vi "Display.vi"(0 "Pressure":dbl=666.0, 1 "InsightMode":T3, 2 "LineOneInfo":T2, 3 "LineTwoInfo":T1, 5 "Temp":string="666", 7 "Angle":dbl=666.0, 9 "Distance":dbl=666.0) -> ()   [LabVIEW 2013]
uses:
  InsightMode.ctl
  LineOneInfo.ctl
  LineTwoInfo.ctl
  <vilib>/Rock Robotics/SystemInterfaces/Typedef/FPGA_TypedefDigitalModule.ctl
  Insight Float Package.vi
  Insight String Package.vi
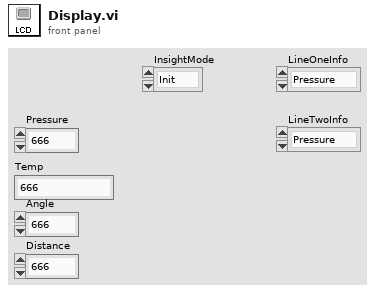
[diagram p1: front panel]
types:
  T1 = typedef "LineTwoInfo.ctl" = enum16{"Pressure", "Temperatue", "Angle", "Distance"}
  T2 = typedef "LineOneInfo.ctl" = enum16{"Pressure", "Temperature", "Angle", "Distance"}
  T3 = typedef "InsightMode.ctl" = enum16{"Init", "Write", "Display", "Disable"}
  T4 = typedef "FPGA_TypedefDigitalModule.ctl" = enum16{"Digital Module 1", "Digital Module 2"}
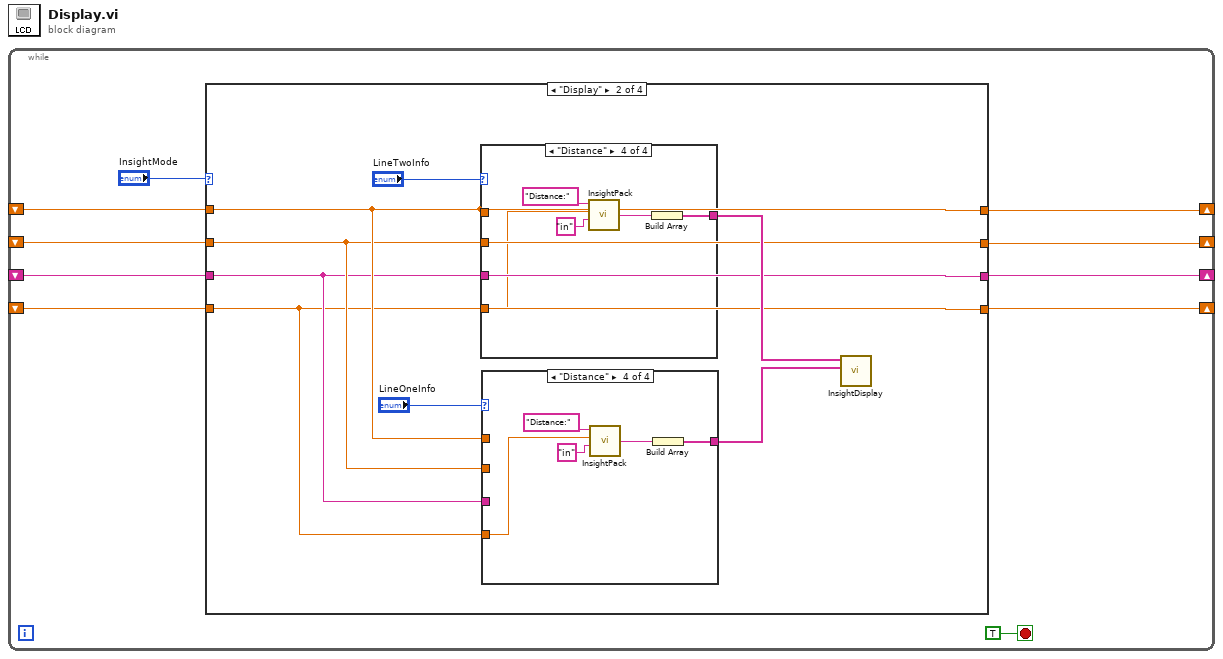
[diagram p0: block diagram]
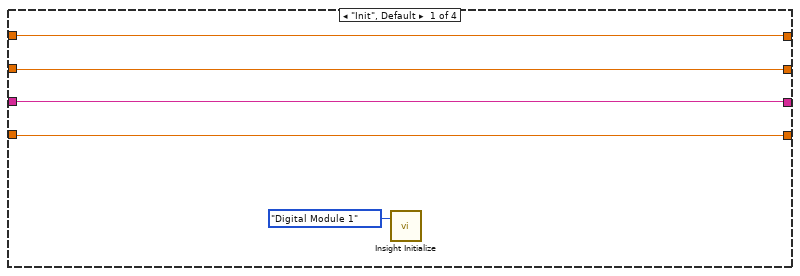
[diagram p2: hidden frame]
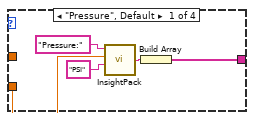
[diagram p3: hidden frame]
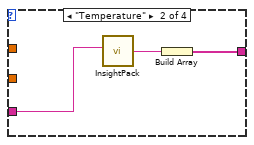
[diagram p4: hidden frame]
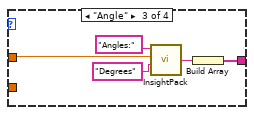
[diagram p5: hidden frame]
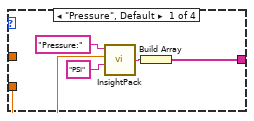
[diagram p6: hidden frame]
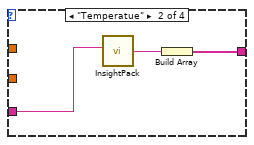
[diagram p7: hidden frame]
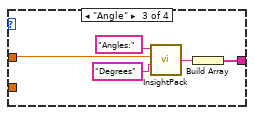
[diagram p8: hidden frame]
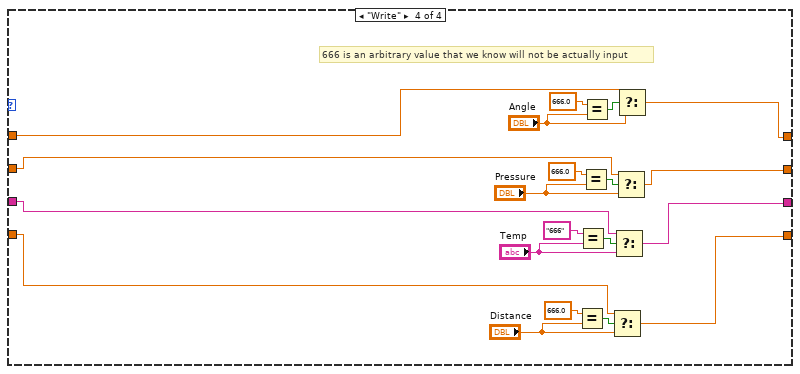
[diagram p10: hidden frame]
diagram:
  n1 = while {
    shift-right: [w6] -> _
    shift-left: _ -> [w5]
    shift-right: [w7] -> _
    shift-left: _ -> [w4]
    shift-right: [w8] -> _
    shift-left: _ -> [w2]
    shift-right: [w9] -> _
    shift-left: _ -> [w3]
    stop <- TRUE stop-if-true
    n2 = case shown="\"Display\"" "InsightMode" {
      tunnel: [w11 w19 w63 w83] -> w6
      tunnel: [w12 w18 w62 w79] -> w7
      tunnel: [w13 w17 w61 w69] -> w8
      tunnel: [w14 w16 w60 w74] -> w9
      tunnel: w5 -> [w11 w19 w63 w82]
      tunnel: w4 -> [w12 w18 w62 w78]
      tunnel: w2 -> [w13 w17 w61 w68]
      tunnel: w3 -> [w14 w16 w60 w73]
      frame "Init", Default {
        n3 = call "Insight Initialize.vi"("Digital Module"=FPGA_TypedefDigitalModule."Digital Module 1") -> ()  [unwired: 2 in]
      }
      frame "Display" {
        n4 = case shown="\"Distance\"" "LineTwoInfo" {
          tunnel: w19 -> [_ _ w52 _]
          tunnel: [w46 w49 w54 w56] -> w20
          tunnel: w18 -> [w44 _ _ _]
          tunnel: w17 -> [_ w48 _ _]
          tunnel: w16 -> [_ _ _ w59]
          frame "Pressure", Default {
            n5 = call-poly "InsightPack.vi"("Footer"="PSI", "Float"=w44, "Header"="Pressure:") -> ("resulting string"=w42:string)  [unwired: 1 in]
            n6 = Build Array(w42) -> (w46:string[])
          }
          frame "Temperatue" {
            n7 = call-poly "InsightPack.vi"("String"=w48) -> ("resulting string"=w47:string)  [unwired: 3 in]
            n8 = Build Array(w47) -> (w49:string[])
          }
          frame "Angle" {
            n9 = call-poly "InsightPack.vi"("Footer"="Degrees", "Float"=w52, "Header"="Angles:") -> ("resulting string"=w53:string)  [unwired: 1 in]
            n10 = Build Array(w53) -> (w54:string[])
          }
          frame "Distance" {
            n11 = call-poly "InsightPack.vi"("Footer"="in", "Float"=w59, "Header"="Distance:") -> ("resulting string"=w55:string)  [unwired: 1 in]
            n12 = Build Array(w55) -> (w56:string[])
          }
        }
        n13 = case shown="\"Distance\"" "LineOneInfo" {
          tunnel: w19 -> [_ _ w34 _]
          tunnel: [w28 w31 w36 w38] -> w21
          tunnel: w18 -> [w26 _ _ _]
          tunnel: w17 -> [_ w30 _ _]
          tunnel: w16 -> [_ _ _ w41]
          frame "Pressure", Default {
            n14 = call-poly "InsightPack.vi"("Footer"="PSI", "Float"=w26, "Header"="Pressure:") -> ("resulting string"=w24:string)  [unwired: 1 in]
            n15 = Build Array(w24) -> (w28:string[])
          }
          frame "Temperature" {
            n16 = call-poly "InsightPack.vi"("String"=w30) -> ("resulting string"=w29:string)  [unwired: 3 in]
            n17 = Build Array(w29) -> (w31:string[])
          }
          frame "Angle" {
            n18 = call-poly "InsightPack.vi"("Footer"="Degrees", "Float"=w34, "Header"="Angles:") -> ("resulting string"=w35:string)  [unwired: 1 in]
            n19 = Build Array(w35) -> (w36:string[])
          }
          frame "Distance" {
            n20 = call-poly "InsightPack.vi"("Footer"="in", "Float"=w41, "Header"="Distance:") -> ("resulting string"=w37:string)  [unwired: 1 in]
            n21 = Build Array(w37) -> (w38:string[])
          }
        }
        n22 = call "InsightDisplay.vi"("Zone 2 Data"=w21, "Zone 1 Data"=w20) -> ()  [unwired: 10 in]
      }
      frame "Disable" {
      }
      frame "Write" {
        # "666 is an arbitrary value that we know will not be actually input"
        n23 = Equal?(x=666.0, y="Distance") -> (x = y?=w70:bool)
        n24 = Equal?(x="666", y="Temp") -> (x = y?=w65:bool)
        n25 = Equal?(x=666.0, y="Pressure") -> (x = y?=w76:bool)
        n26 = Equal?(x=666.0, y="Angle") -> (x = y?=w64:bool)
        n27 = Select(t=w73, s=w70, f="Distance") -> (s? t:f=w74:dbl)
        n28 = Select(t=w68, s=w65, f="Temp") -> (s? t:f=w69:string)
        n29 = Select(t=w78, s=w76, f="Pressure") -> (s? t:f=w79:dbl)
        n30 = Select(t=w82, s=w64, f="Angle") -> (s? t:f=w83:dbl)
      }
    }
  }
